vi "Set Item Resource String.vi"(7 "ItemName (ASCII)":string, 8 "error in (no error)":errorcluster, 9 "Text (UTF-16)":string, 10 "Language":i32, 11 "GObject in":refnum<class "GObject.lvclass">) -> (0 "error out":errorcluster, 3 "GObject out":refnum<class "GObject.lvclass">)   [LabVIEW 2013, in "SET Project Data.lvlib" / "GObject.lvclass"]
uses:
  GObject.lvclass
  GObject.lvclass/GObject.ctl
  Resource Data Class/Resource Data.lvclass
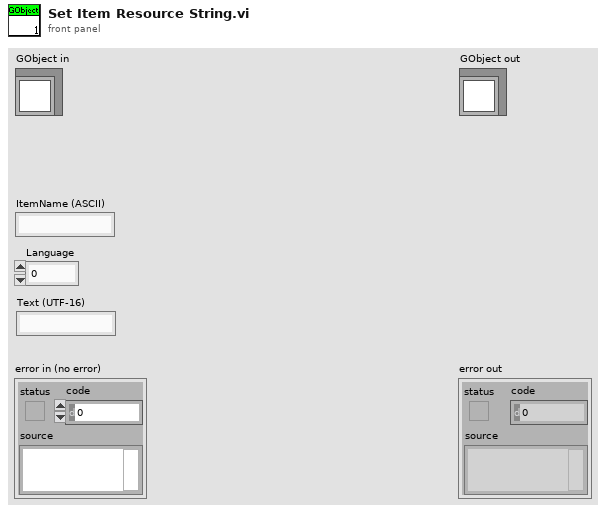
[diagram p1: front panel]
types:
  T1 = typedef "SET Project Data.lvlib/ProjFile_Resource Entry.ctl" = cluster{"RID":string, "Tag":string, "Strings [] (UTF-16)":string[], "Shared?":bool}
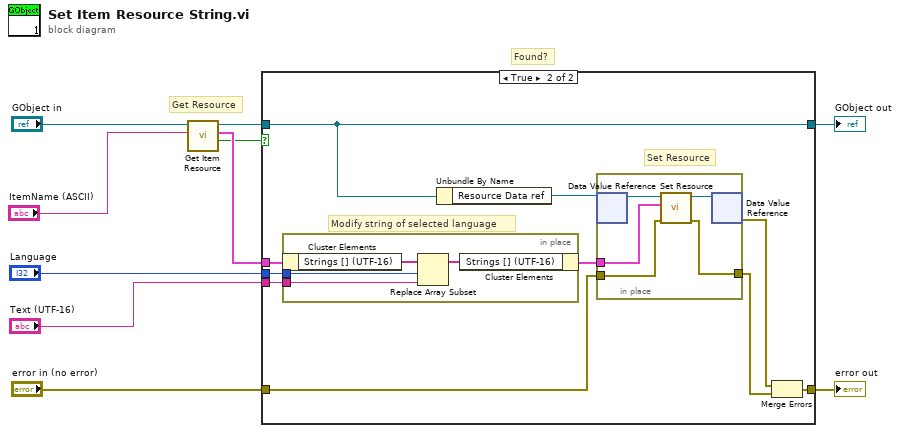
[diagram p0: block diagram]
diagram:
  # "Found?"
  # "Get Resource"
  n1 = call "Get Item Resource.vi"("ItemName"="ItemName (ASCII)", "GObject in"="GObject in") -> ("Found?"=w4:bool, "Resource"=w8:T1, "GObject out"=w5:refnum<class "GObject.lvclass">)  [unwired: 5 in, 2 out]
  n2 = case shown="True" w4 {
    tunnel: w8 -> [_ w21]
    tunnel: "Language" -> [_ w20]
    tunnel: "Text (UTF-16)" -> [_ w19]
    tunnel: w5 -> [w12 w17]
    tunnel: [w12 w17] -> w3
    tunnel: "error in (no error)" -> [w11 w16]
    tunnel: [w11 w13] -> w1
    frame False {
    }
    frame True {
      # "Modify string of selected language"
      # "Set Resource"
      n3 = in-place {
        in-place-border: w20 -> [w24]
        in-place-border: w19 -> [w23]
        n4 = in-place-cluster #1(w21) -> ("Strings [] (UTF-16)"=w26:string[])
        n5 = Replace Array Subset(array=w26, new element=w23, index=w24) -> (w25:string[])
        n6 = in-place-cluster #1("Strings [] (UTF-16)"=w25) -> (w18:T1)
      }
      n7 = Unbundle By Name(w17) -> ("Resource Data ref"=w22:refnum<data-value>)
      n8 = in-place {
        in-place-border: w18 -> [w30]
        in-place-border: w16 -> [w28]
        in-place-border: [w27] -> w14
        n9 = in-place-dvr #2(w22) -> (w31:refnum<class "Resource Data.lvclass">)  [unwired: 1 out]
        n10 = call "Set Resource.vi"("error in (no error)"=w28, "Resource"=w30, "LangFile in"=w31) -> ("error out"=w27:errorcluster, "LangFile out"=w29:refnum<class "Resource Data.lvclass">)  [unwired: 7 in]
        n11 = in-place-dvr #2(w29) -> (w15:errorcluster)  [unwired: 1 out]
      }
      n12 = Merge Errors(w15, w14) -> (w13:errorcluster)
    }
  }
  "error out" <- w1
  "GObject out" <- w3
